vi "Generate Signal.vi"(7 "settings.<user name>":T4, 8 "register bus":T2={"Speed"="Speed", "Crank Angle"="Crank Angle", "Cycle Angle"="Cycle Angle", "Crank Count"="Crank Count", "Cycle Count"="Cycle Count", "1.25 MHz Counter"="1.25 MHz Counter", "Crank Rollover"="Crank Rollover", "Cycle Rollover"="Cycle Rollover", "shared settings"={"start"=0.0, "stuck limit"=0.0}} {"shared settings"."start" format="%#.15g"}, 10 "triggered knock data":T5[](array[typedef]), 11 "input.<user name>":T1) -> (3 "knock signal":i16)   [LabVIEW 2013, in "Engine Simulation Toolkit.lvlib" / "Knock Sensor.lvlib"]
doc: "Creates a base frequency sinewave continously based upon a user specified frequency, or upon engine speed. Adds high frequency noise on top of the base frequency when a cylinder knock is triggered.\n\n<b>settings.<user name></b> - settings for the component. NI VeriStand will set these values. Create a control for this input. Replace <user name> with the name you wish this component to display as inside NI VeriStand. Make this name consistent for all controls, indicators, for all VIs of this component.\n<b>input.<user name></b> - input for the component. NI VeriStand will set these values. Create a control for this input. Replace <user name> with the name you wish this component to display as inside NI VeriStand. Make this name consistent for all controls, indicators, for all VIs of this component.\n<b>triggered knock data</b> - data about the cylinder's knock status sent to the Generate Signal.vi\n<b>register bus</b> - connect this input to the output of the initialize APU VI. This contains references to APU state variables like position and speed.\n\n<b>knock signal</b> - analog knock signal. wire this to an analog output IO node"
uses:
  Knock Sensor.lvlib
  Triggered Cylinder Data.ctl
  Generate Settings.ctl
  APU/Register Bus.ctl
  APU/Shared Settings.ctl
  Generate Input.ctl
  <vilib>/Platform/TimedLoop/XDataNode/timing_clust.ctl
  <vilib>/Platform/TimedLoop/XDataNode/nitl_modes.ctl
  <vilib>/Platform/TimedLoop/XDataNode/wakeup.ctl
  <vilib>/rvi/Emulation/niFpgaSctlEmulationGetInTimedLoop.vi
  <vilib>/rvi/Emulation/niFpgaEmulationReportErrorSimple.vi
  <vilib>/rvi/Emulation/niFpgaGetClockAttributes.vi
  <vilib>/rvi/Emulation/niFpgaCriticalErrorInLSC.vi
  <vilib>/rvi/DataTransferAndStorage/Container/Common/niFpgaContainerExecOnDevCompGetState.vi
  <vilib>/rvi/DataTransferAndStorage/Register/Emulation/niFpgaRegisterEmulationFpgaImpl.vi
  <instcachedir>/0/niFpgaRegisterEmulationFpgaImpl_DCF4BC0110594B98B44A971D60CEEC4D.lvgen/niFpgaRegisterEmulationFpgaImpl_DCF4BC0110594B98B44A971D60CEEC4D_005.vi
  <vilib>/rvi/DataTransferAndStorage/Container/Common/niFpgaContainerGetUniqueNameForEmu.vi
  <instcachedir>/0/niFpgaRegisterEmulationFpgaImpl_DCF4BC0110594B98B44A971D60CEEC4D.lvgen/niFpgaRegisterEmulationFpgaImpl_DCF4BC0110594B98B44A971D60CEEC4D_018.vi
  <vilib>/Platform/TimedLoop/XDataNode/XDataNode.xnode
  <vilib>/rvi/DataTransferAndStorage/Container/XNode/niFpgaContainer.xnode
  <vilib>/rvi/DataTransferAndStorage/Register/Emulation/niFpgaRegisterEmulationRefIn.vi
  <vilib>/Platform/TimedLoop/XDataNode/XDNodeRunTimeDep.lvlib
  APU/APU.lvlib
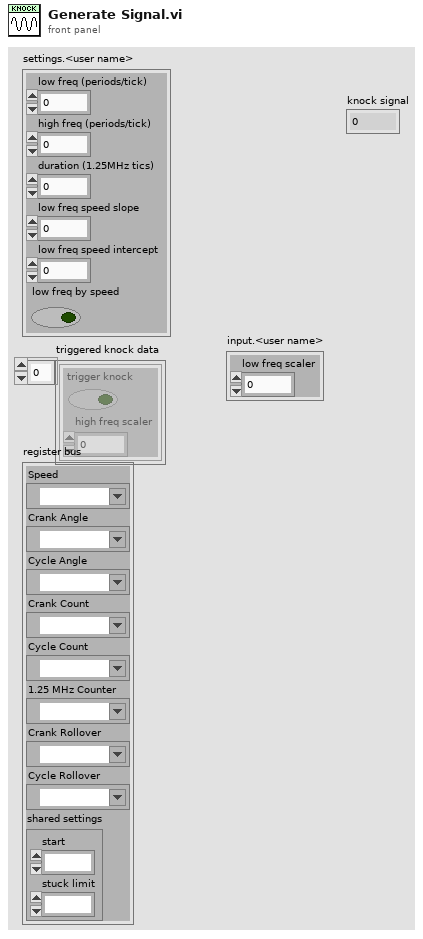
[diagram p1: front panel]
types:
  T1 = typedef "Engine Simulation Toolkit.lvlib/Knock Sensor.lvlib/Generate Input.ctl" = cluster{"low freq scaler":fxp<+,10,0>}
  T2 = typedef "Engine Simulation Toolkit.lvlib/APU.lvlib/Register Bus.ctl" = cluster{"Speed":refnum<k21>, "Crank Angle":refnum<k21>, "Cycle Angle":refnum<k21>, "Crank Count":refnum<k21>, "Cycle Count":refnum<k21>, "1.25 MHz Counter":refnum<k21>, "Crank Rollover":refnum<k21>, "Cycle Rollover":refnum<k21>, "shared settings":T3}
  T3 = typedef "Engine Simulation Toolkit.lvlib/APU.lvlib/Shared Settings.ctl" = cluster{"start":fxp<+,17,17>, "stuck limit":fxp<+,18,18>}
  T4 = typedef "Engine Simulation Toolkit.lvlib/Knock Sensor.lvlib/Generate Settings.ctl" = cluster{"low freq (periods/tick)":fxp<+,32,0>, "high freq (periods/tick)":fxp<+,32,0>, "duration (1.25MHz tics)":fxp<+,18,18>, "low freq speed slope":fxp<+,16,-3>, "low freq speed intercept":fxp<+,10,-10>, "low freq by speed":bool}
  T5 = typedef "Engine Simulation Toolkit.lvlib/Knock Sensor.lvlib/Triggered Cylinder Data.ctl" = cluster{"trigger knock":bool, "high freq scaler":fxp<+,10,0>}
  T6 = typedef "XDNodeRunTimeDep.lvlib/timing_clust.ctl" = cluster{"Expected End [f-1]":u64, "Actual End [f-1]":u64, "Finished Late? [f-1]":bool, "Expected End [i-1]":u64, "Actual End [i-1]":u64, "Finished Late? [i-1]":bool, "Expected Start [i]":u64, "Actual Start [i]":u64, "Expected Start [f]":u64, "Actual Start [f]":u64, "Source Name":string, "Structure Name":string, "Period":i64, "Deadline":i64, "Offset":i64, "Start":i64, "Priority":i32, "Timeout":i32, "Mode":T7, "Wakeup Reason":T8, "Error":errorcluster, "Source Type":string, "Secondary Source Type":string, "Global End Time":u64, "Global Start Time":u64, "Frame Duration":u64, "Iteration Duration":u64, "Assigned CPU":i32, "I/O Scan Engine Mode":u32}
  T7 = typedef "XDNodeRunTimeDep.lvlib/nitl_modes.ctl" = enum32{"No Change", "Process missed periods, maintain original phase", "Discard missed periods, maintain original phase", "Process missed periods, ignore original phase", "Discard missed periods, ignore original phase"}
  T8 = typedef "XDNodeRunTimeDep.lvlib/wakeup.ctl" = enum32{"Normal", "Aborted", "Asynchronous wakeup", "Timing source error", "Timed loop error", "Timeout"}
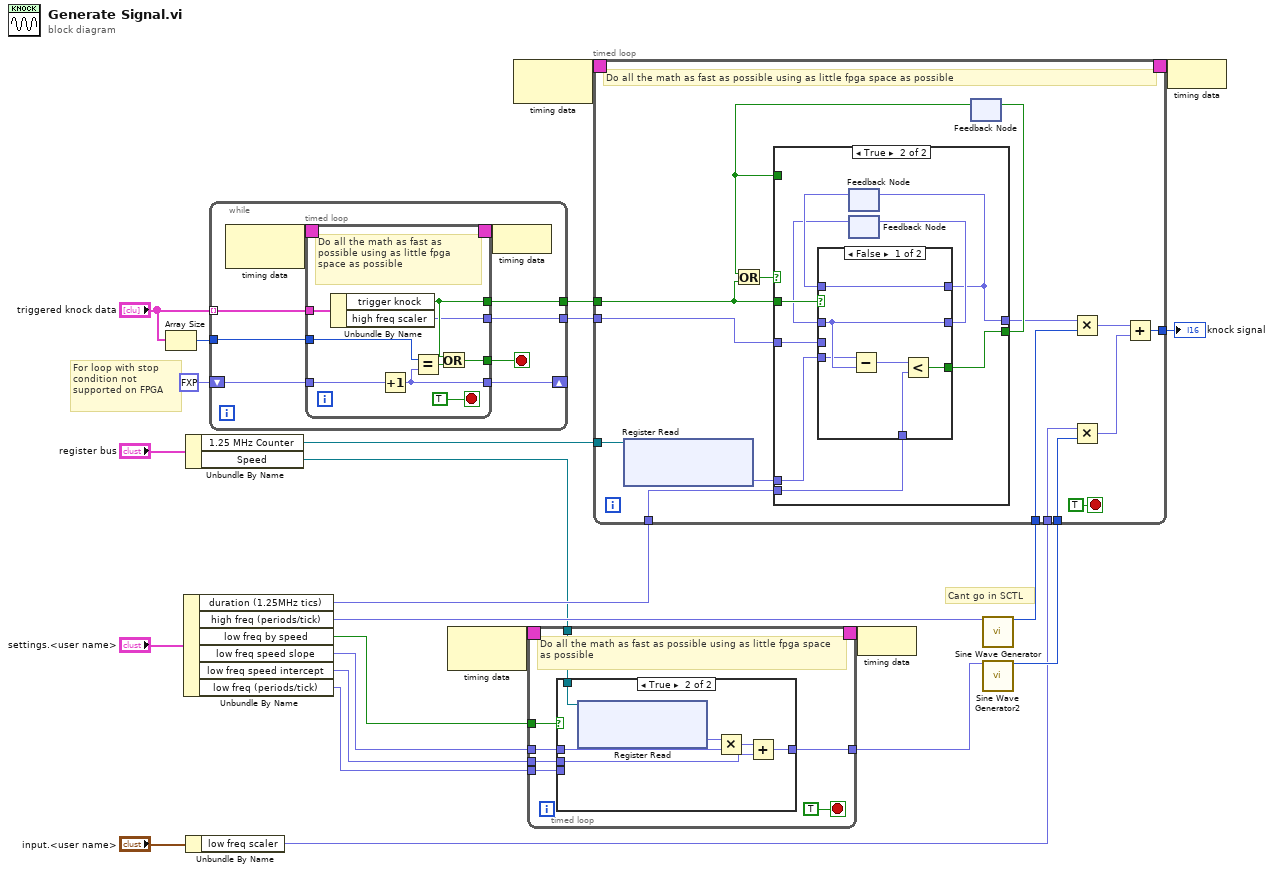
[diagram p0: block diagram]
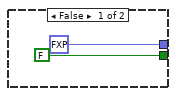
[diagram p3: hidden frame]
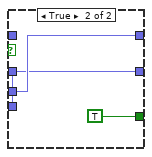
[diagram p4: hidden frame]
diagram:
  # "For loop with stop condition not supported on FPGA"
  # "Cant go in SCTL"
  n1 = Array Size(array="triggered knock data") -> (size(s)=w18:i32)
  n2 = Unbundle By Name("settings.<user name>") -> ("duration (1.25MHz tics)"=w24:fxp<+,18,18>, "high freq (periods/tick)"=w16:fxp<+,32,0>, "low freq by speed"=w6:bool, "low freq speed slope"=w4:fxp<+,16,-3>, "low freq speed intercept"=w3:fxp<+,10,-10>, "low freq (periods/tick)"=w1:fxp<+,32,0>)
  n3 = Unbundle By Name("register bus") -> ("1.25 MHz Counter"=w22:refnum<k21>, "Speed"=w5:refnum<k21>)
  n4 = Unbundle By Name("input.<user name>") -> ("low freq scaler"=w9:fxp<+,10,0>)
  n5 = while {
    tunnel: "triggered knock data" -> [w34] mode=indexing
    tunnel: [w33] -> w21
    tunnel: [w32] -> w20
    tunnel: w18 -> [w28]
    shift-right: [w29] -> _
    shift-left: fxp<+,5,5> 0.0 -> [w30]
    stop <- w31 stop-if-true
    n6 = node-c288() -> (w27:T6)  [unwired: 1 in]
    n7 = timed-loop {
      timing: w27 -> [_]
      timing-out: [_] -> w26
      tunnel: w34 -> [w43]
      tunnel: [w42] -> w33
      tunnel: [w41] -> w32
      tunnel: [w40] -> w31
      tunnel: w30 -> [w39]
      tunnel: [w38] -> w29
      tunnel: w28 -> [w37]
      stop <- TRUE stop-if-true
      # "Do all the math as fast as possible using as little fpga space as possible"
      n8 = Unbundle By Name(w43) -> ("trigger knock"=w42:bool, "high freq scaler"=w41:fxp<+,10,0>)
      n9 = Increment(x=w39) -> (x+1=w38:fxp<+,5,5>)
      n10 = Equal?(x=w37, y=w38) -> (x = y?=w36:bool)
      n11 = Or(x=w42, y=w36) -> (x .or. y?=w40:bool)
    }
    n12 = node-c288(w26) -> ()
  }
  n13 = node-c288() -> (w8:T6)  [unwired: 1 in]
  n14 = node-c288() -> (w15:T6)  [unwired: 1 in]
  n15 = timed-loop {
    timing: w8 -> [_]
    timing-out: [_] -> w7
    tunnel: w6 -> [w53]
    tunnel: w5 -> [w52]
    tunnel: w4 -> [w51]
    tunnel: w3 -> [w50]
    tunnel: [w49] -> w2
    tunnel: w1 -> [w48]
    stop <- TRUE stop-if-true
    # "Do all the math as fast as possible using as little fpga space as possible"
    n16 = case shown="True" w53 {
      tunnel: w52 -> [_ w61]
      tunnel: w51 -> [_ w59]
      tunnel: w50 -> [_ w57]
      tunnel: [w55 w56] -> w49
      tunnel: w48 -> [w55 _]
      frame False {
      }
      frame True {
        n17 = xnode ("Register Read")("Register In"=w61) -> ("Data"=w60:fxp<+/-,23,2>)  [unwired: 1 out]
        n18 = Multiply(x=w60, y=w59) -> (x*y=w58:fxp<+,32,0>)
        n19 = Add(x=w58, y=w57) -> (x+y=w56:fxp<+,32,0>)
      }
    }
  }
  n20 = node-c288(w7) -> ()
  n21 = call "Sine Wave Generator"("frequency (periods/tick)"=w16) -> ("sine out"=w13:i16)  [unwired: 14 in]
  n22 = call "Sine Wave Generator2"("frequency (periods/tick)"=w2) -> ("sine out"=w12:i16)  [unwired: 14 in]
  n23 = timed-loop {
    timing: w15 -> [_]
    timing-out: [_] -> w14
    tunnel: w24 -> [w79]
    tunnel: w22 -> [w75]
    tunnel: w21 -> [w73]
    tunnel: w20 -> [w72]
    tunnel: w13 -> [w67]
    tunnel: w9 -> [w66]
    tunnel: w12 -> [w65]
    tunnel: [w64] -> w11
    stop <- TRUE stop-if-true
    # "Do all the math as fast as possible using as little fpga space as possible"
    n24 = xnode ("Register Read")("Register In"=w75) -> ("Data"=w74:fxp<+,18,18>)  [unwired: 1 out]
    n25 = feedback #1() -> (w77:bool)  [unwired: 1 in]
    n26 = Or(x=w77, y=w73) -> (x .or. y?=w78:bool)
    n27 = case shown="True" w78 {
      tunnel: w73 -> [_ w90]
      tunnel: w77 -> [_ _]
      tunnel: [fxp<+,1,1> 0.0 w82] -> w68
      tunnel: [FALSE w88] -> w76
      tunnel: w79 -> [_ w87]
      tunnel: w72 -> [_ w86]
      tunnel: w74 -> [_ w83]
      frame False {
      }
      frame True {
        n28 = feedback #2() -> (w89:fxp<+,10,0>)  [unwired: 1 in]
        n29 = feedback #3() -> (w84:fxp<+,18,18>)  [unwired: 1 in]
        n30 = case shown="False" w90 {
          tunnel: [w96 w98] -> w82
          tunnel: w89 -> [w96 _]
          tunnel: [w94 TRUE] -> w88
          tunnel: w87 -> [w95 _]
          tunnel: w86 -> [_ w98]
          tunnel: [w93 w97] -> w85
          tunnel: w84 -> [w93 _]
          tunnel: w83 -> [w91 w97]
          frame False {
            n31 = Subtract(x=w91, y=w93) -> (x-y=w92:fxp<+,18,18>)
            n32 = Less?(x=w92, y=w95) -> (x < y?=w94:bool)
          }
          frame True {
          }
        }
        n33 = feedback-in #2(w82) -> ()
        n34 = feedback-in #3(w85) -> ()
      }
    }
    n35 = feedback-in #1(w76) -> ()
    n36 = Multiply(x=w68, y=w67) -> (x*y=w70:fxp<+/-,18,16>)
    n37 = Multiply(x=w66, y=w65) -> (x*y=w69:fxp<+/-,18,16>)
    n38 = Add(x=w70, y=w69) -> (x+y=w64:i16)
  }
  "knock signal" <- w11
  n39 = node-c288(w14) -> ()
